vi "Channel Initialize.vi"(0 "Item Ref in":T1 format="%.0x", 7 "error in (no error)":errorcluster) -> (14 "Default Value":dbl, 16 "Unit ID":u8, 17 "Sub-Index (Bool)":u16, 18 "Registers":i32, 19 "input?":bool, 20 "Channel Ref out":T1 format="%.0x", 21 "Name":string, 22 "Description":string, 23 "Starting Address":u16, 24 "DataType":T2, 25 "Valid?":bool, 26 "Status Message":string, 27 "error out":errorcluster)   [LabVIEW 2021, in "Modbus Master System Explorer.lvlib"]
uses:
  Modbus Master System Explorer.lvlib
  Shared/Controls/Data Model/DataType.ctl
  <vilib>/NI VeriStand/Custom Device API/Custom Device Item Ref.ctl
  <vilib>/NI VeriStand/Custom Device API/Custom Device API.lvlib
  Shared/Modbus Master Shared.lvlib
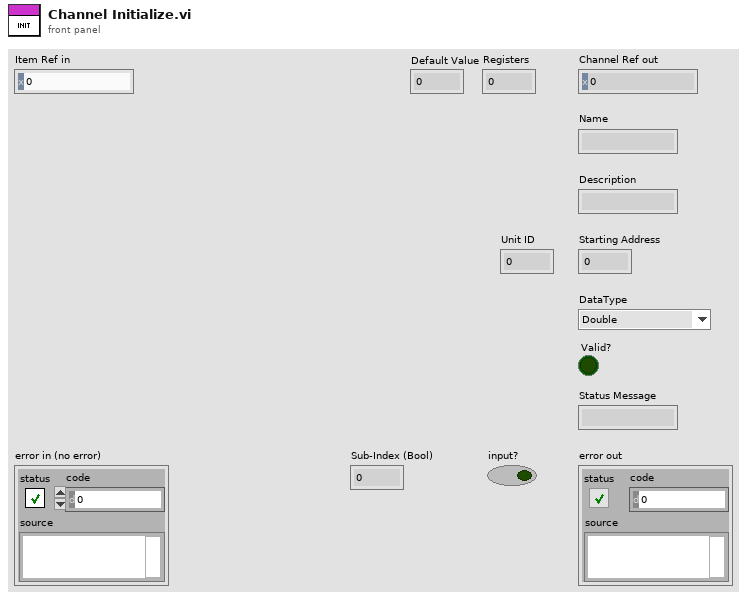
[diagram p1: front panel]
types:
  T1 = typedef "Custom Device API.lvlib/Custom Device Item Ref.ctl" = u64
  T2 = typedef "Modbus Master Shared.lvlib/DataType.ctl" = enum16{"Double", "Single", "I64", "I32", "I16", "I8", "U64", "U32", "U16", "U8", "Boolean"}
  T3 = typedef "Custom Device API.lvlib/Custom Device Item Info.ctl" = cluster{"Name":string, "Is Channel":bool, "GUID":string, "Is Waveform":bool}
  T4 = typedef "Modbus Master Shared.lvlib/Mapping.ctl" = cluster{"DataType":T2, "Unit ID":u8, "Starting Address":u16, "Sub-Index (Bool)":u16, "VS Reference":T1}
  T5 = typedef "Custom Device API.lvlib/Custom Device Channel.ctl" = cluster{"Type":T6, "Units":string, "Default Value":dbl, "Faultable":bool, "Scalable":bool}
  T6 = typedef "Custom Device API.lvlib/Custom Device Channel Type.ctl" = enum16{"Input", "Output"}
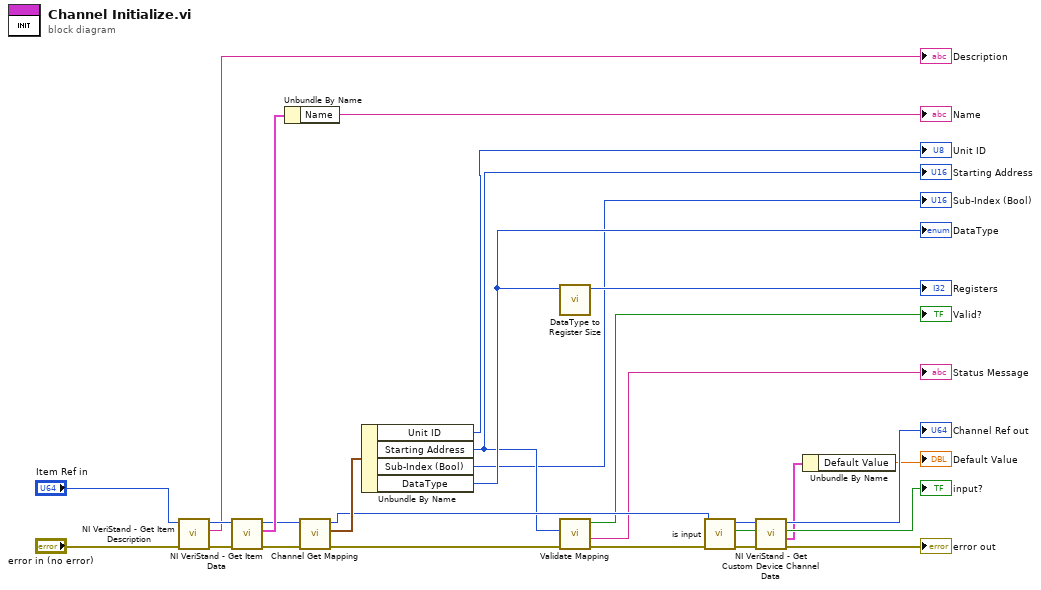
[diagram p0: block diagram]
diagram:
  n1 = call <vilib>:"NI VeriStand - Get Item Description.vi"("error in (no error)"="error in (no error)", "Item Ref in"="Item Ref in") -> ("error out"=w26:errorcluster, "Description"=→"Description":string, "Item Ref out"=w27:T1)  [unwired: 7 out]
  n2 = call <vilib>:"NI VeriStand - Get Item Data.vi"("error in (no error)"=w26, "Item Ref in"=w27) -> ("error out"=w23:errorcluster, "Item Info"=w25:T3, "Item Ref out"=w24:T1)  [unwired: 7 out]
  n3 = Unbundle By Name(w25) -> ("Name"=→"Name":string)
  n4 = call "Channel Get Mapping.vi"("error in (no error)"=w23, "Item Ref in"=w24) -> ("error out"=w20:errorcluster, "Mapping"=w22:T4, "Item Ref out"=w21:T1)  [unwired: 7 in]
  n5 = Unbundle By Name(w22) -> ("Unit ID"=→"Unit ID":u8, "Starting Address"=w10:u16, "Sub-Index (Bool)"=→"Sub-Index (Bool)":u16, "DataType"=w11:T2)
  "Starting Address" <- w10
  "DataType" <- w11
  n6 = call "DataType to Register Size.vi"("DataType"=w11) -> ("Registers"=→"Registers":i32)  [unwired: 9 in, 1 out]
  n7 = call "Validate Mapping.vi"("error in (no error)"=w20, "Mapping"=w10) -> ("error out"=w19:errorcluster, "Status Message"=→"Status Message":string, "Valid?"=→"Valid?":bool)  [unwired: 7 in]
  n8 = call "is input.vi"("error in (no error)"=w19, "Item Ref in"=w21) -> ("error out"=w6:errorcluster, "input?"=→"input?":bool, "Channel Ref out"=w7:T1)  [unwired: 7 in]
  n9 = call <vilib>:"NI VeriStand - Get Custom Device Channel Data.vi"("error in (no error)"=w6, "Channel Ref in"=w7) -> ("error out"=→"error out":errorcluster, "Channel"=w3:T5, "Channel Ref out"=→"Channel Ref out":T1)  [unwired: 4 in, 3 out]
  n10 = Unbundle By Name(w3) -> ("Default Value"=→"Default Value":dbl)
